vi "RPM Ready.vi"(8 "Right RPM Target":dbl, 9 "Left RPM Target":dbl, 10 "Right RPM":dbl, 11 "Left RPM":dbl) -> (3 "RPM gud?":bool)   [LabVIEW 2016]
uses:
  Robot Global Data.vi
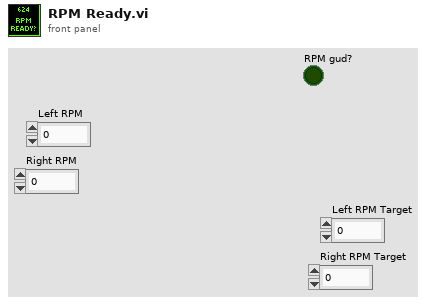
[diagram p1: front panel]
types:
  T1 = typedef "Dashboard Control Data.ctl" = cluster{"Drivetrain Settings":T2, "Intake Presets ":T3, "Shooter Presets":T4}
  T2 = typedef "Drivetrain Settings.ctl" = cluster{"Gyro Tolerance":dbl}
  T3 = typedef "Intake Presets.ctl" = cluster{"Intake Speed ":dbl, "Outake Speed":dbl, "Set Time":dbl}
  T4 = typedef "Shooter Presets.ctl" = cluster{"Key Shot":cluster{"Left ":dbl, "Right":dbl, "Angle":dbl}, "Distance Shot":cluster{"Left":dbl, "Right":dbl, "Angle":dbl}, "RPM Tolerance":dbl}
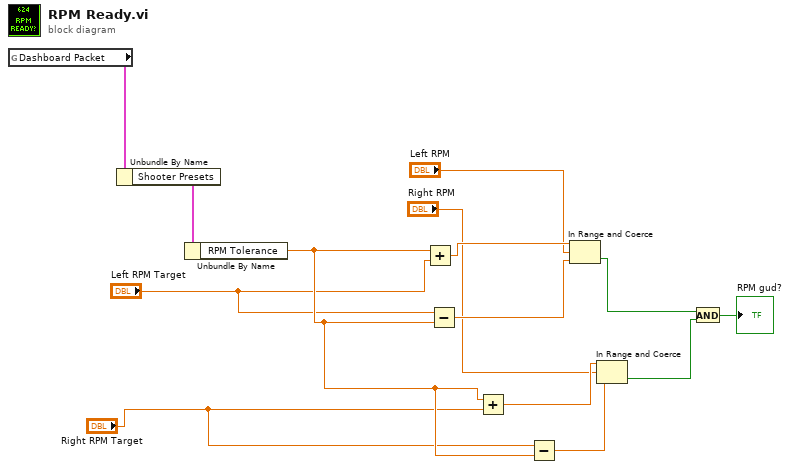
[diagram p0: block diagram]
diagram:
  n1 = global read "Robot Global Data.vi" "Dashboard Packet"() -> (w11:T1)
  n2 = Unbundle By Name(w11) -> ("Shooter Presets"=w10:T4)
  n3 = Unbundle By Name(w10) -> ("RPM Tolerance"=w9:dbl)
  n4 = Add(x=w9, y="Left RPM Target") -> (x+y=w6:dbl)
  n5 = Subtract(x="Left RPM Target", y=w9) -> (x-y=w5:dbl)
  n6 = Add(x=w9, y="Right RPM Target") -> (x+y=w4:dbl)
  n7 = Subtract(x="Right RPM Target", y=w9) -> (x-y=w3:dbl)
  n8 = In Range and Coerce(upper limit=w6, x="Left RPM", lower limit=w5) -> (In Range?=w13:bool)  [unwired: 1 out]
  n9 = In Range and Coerce(upper limit=w4, x="Right RPM", lower limit=w3) -> (In Range?=w14:bool)  [unwired: 1 out]
  n10 = And(x=w13, y=w14) -> (x .and. y?=→"RPM gud?":bool)
